vi "execute-mark-frame.vi"(6 "Coords":T1, 7 "This VI":refnum<vi>, 8 "error in (no error)":errorcluster, 9 "frame.name":string, 10 "symbol":i32) -> (0 "error out":errorcluster, 1 "ok":bool, 2 "action":T2)   [LabVIEW 2015]
uses:
  subs/frame.type.ctl
  <vilib>/Utility/miscctls.llb/LVPoint32TypeDef.ctl
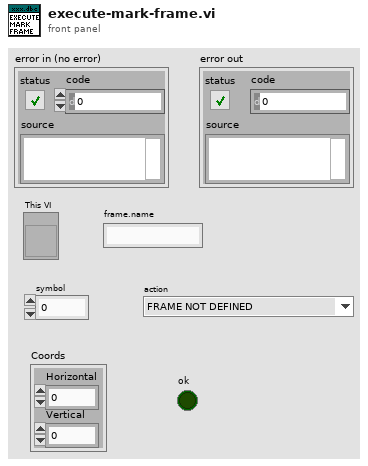
[diagram p1: front panel]
types:
  T1 = typedef "LVPoint32TypeDef.ctl" = cluster{"Horizontal":i32, "Vertical":i32}
  T2 = typedef "frame.type.ctl" = enum16{"FRAME NOT DEFINED", "DUT OUTPUT FRAME", "DUT INPUT FRAME"}
  T3 = typedef "LVRectTypeDef.ctl" = cluster{"Left":i16, "Top":i16, "Right":i16, "Bottom":i16}
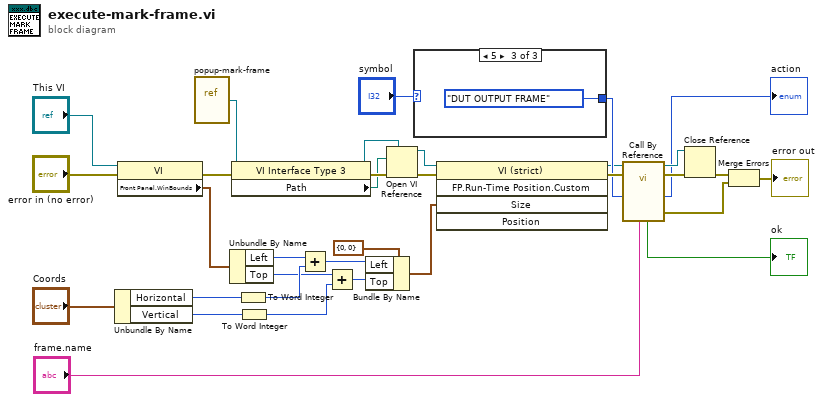
[diagram p0: block diagram]
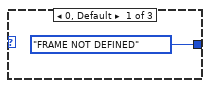
[diagram p2: hidden frame]
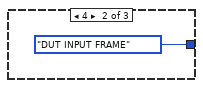
[diagram p3: hidden frame]
diagram:
  n1 = Unbundle By Name("Coords") -> ("Horizontal"=w16:i32, "Vertical"=w17:i32)
  n2 = property class="VI"(reference="This VI", error in="error in (no error)") -> (error out=w19:errorcluster, "Front Panel.WinBounds"=w15:T3)  [unwired: 1 out]
  n3 = vi-ref "popup-mark-frame.vi"() -> (w32:refnum<vi>)
  n4 = Unbundle By Name(w15) -> ("Left"=w14:i16, "Top"=w12:i16)
  n5 = property class="VI Interface Type 3"(reference=w32, error in=w19) -> (reference out=w31:refnum<vi>, error out=w29:errorcluster, "Path"=w4:path)
  n6 = To Word Integer(number=w16) -> (16bit integer=w13:i16)
  n7 = To Word Integer(number=w17) -> (16bit integer=w11:i16)
  n8 = Add(x=w14, y=w13) -> (x+y=w8:i16)
  n9 = Add(x=w12, y=w11) -> (x+y=w7:i16)
  n10 = Bundle By Name(cluster=cluster{"Top":i16, "Left":i16} {"Top"=0, "Left"=0} ("Position"), "Left"=w8, "Top"=w7) -> (w9:cluster{"Top":i16, "Left":i16})
  n11 = Open VI Reference(type specifier VI Refnum (for type only)=w31, vi path=w4, error in (no error)=w29) -> (vi reference=w5:refnum<vi>, error out=w6:errorcluster)  [unwired: 3 in]
  n12 = case shown="5" "symbol" {
    tunnel: [frame.type."FRAME NOT DEFINED" ("frame.type") frame.type."DUT INPUT FRAME" ("frame.type") frame.type."DUT OUTPUT FRAME" ("frame.type")] -> w25
    frame 0, Default {
    }
    frame 4 {
    }
    frame 5 {
    }
  }
  n13 = invoke class="VI (strict)" method="FP.Run-Time Position.Custom"(reference=w5, error in=w6, "Size"=w9) -> (reference out=w3:refnum<vi>, error out=w33:errorcluster)  [unwired: 2 in, 3 out]
  n14 = call-by-ref "?"(reference=w3, error in=w33, "frame.name"="frame.name", "frame.type.in"=w25) -> (reference out=w26:refnum<vi>, error out=w27:errorcluster, 0:"error out"=w22:errorcluster, "grame.type.out"=→"action":T2, "ok 2"=→"ok":bool)  [unwired: 7 in]
  n15 = Close Reference(reference=w26, error in (no error)=w27) -> (error out=w28:errorcluster)
  n16 = Merge Errors(w28, w22) -> (→"error out":errorcluster)
